vi "Z6_Beamline.ProcCases.vi"(0 "i ref in":refnum<vi>, 1 "selector":string, 2 "Data":T1, 3 "call cluster":T2={"Object"="", "Selector"="", "CallType"=enum."synchronous", "Async Object"="", "Async Selector"="", "Data Descriptor"="", "Data"=[], "Error #"=0, "Expire"=0}, 5 "error in (no error)":errorcluster) -> (14 "i ref out":refnum<vi>, 17 "answer cluster":T2={"Object"="", "Selector"="", "CallType"=enum."synchronous", "Async Object"="", "Async Selector"="", "Data Descriptor"="", "Data"=[], "Error #"=0, "Expire"=0}, 19 "error out":errorcluster)   [LabVIEW 2014, in "Z6_Beamline.lvlib"]
doc: "This method is called by a process from within the default case in the event loop. The methods of a class that are linked to events will be called from THIS method. Add your code here."
uses:
  Z6_Beamline.lvlib
  CSCore/CSSystem/CoreDefs/CoreDefs.call_type.ctl
  CSCore/BaseProcess/BaseProcess.descriptor string definition.ctl
  CSCore/CSSystem/CoreDefs/CoreDefs.rawDataType.ctl
  CSCore/CSSystem/CoreLib/CoreLib.string 2 byte array.vi
  CSCore/BaseProcess/BaseProcess.lvlib
  CSCore/CAEObj/CAEObj.lvlib
  CSCore/CSSystem/CoreLib/CoreLib.lvlib
  PH_BL-Master/PH_BL-Master.lvlib
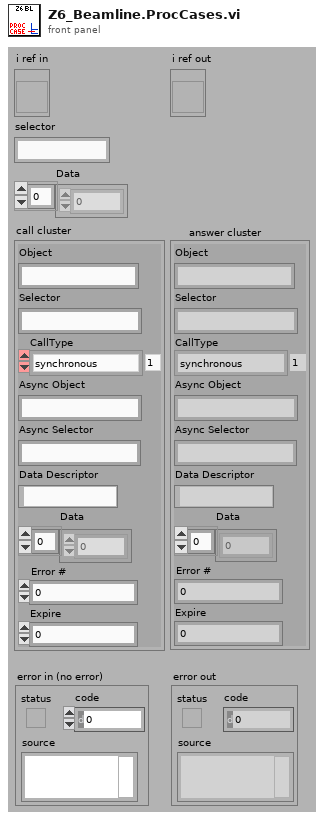
[diagram p1: front panel]
types:
  T1 = typedef "CoreDefs.rawDataType.ctl" = i8[]
  T2 = typedef "CoreDefs.call_type.ctl" = cluster{"Object":string, "Selector":string, "CallType":enum16{"simple", "synchronous", "asynchronous"}, "Async Object":string, "Async Selector":string, "Data Descriptor":T3, "Data":T1, "Error #":i32, "Expire":u32}
  T3 = typedef "BaseProcess.lvlib/BaseProcess.descriptor string definition.ctl" = string
  T4 = typedef "PH_BL-Master.lvlib/PH_BL-Master.i attribute.ctl" = cluster{"Remote controlled":bool, "Boolean Condition Service Subscriber":refnum<vi>[], "Picture Condition Service Subscriber":refnum<vi>[], "R2S":cluster{"GUI Ref":refnum<vi>, "State":bool}, "Vacua":cluster{"GUI Ref":refnum<vi>, "Limit":dbl, "Curr Value":dbl, "in range":bool}[], "O2 Inspection":cluster{"GUI Ref":refnum<vi>, "Concentration":dbl, "State":T5}[], "Boolean Status Service Subscriber":cluster{"GUI Ref":refnum<vi>, "Status":T5, "no Link?":bool, "Status Subscriber Class":T6}[], "Picture Status Service Subscriber":cluster{"GUI Ref":refnum<vi>, "Status":T5, "no Link?":bool, "Status Subscriber Class":T6}[], "6P 4Q Service Subscriber":cluster{"GUI Ref":refnum<vi>, "Selector":T7, "no Link?":bool}[], "Index of latest 6P 4Q changing Instance":i32, "Index of latest Picture Status changing Instance":i32, "Index of latest Boolean Status changing Instance":i32, "Vision ID on same Node":string, "Start Phase over?":bool, "GUI Ref Delete":refnum<vi>}
  T5 = typedef "PH_StatusHandler.lvlib/PH_StatusHandler.Status.ctl" = i16
  T6 = typedef "PH_BL-Master.lvlib/PH_BL-Master.Status Subscriber Class.ctl" = enum16{"unknown", "Switch", "BB", "6P Switch", "Switch GUI", "Switch and 6P State", "Force Sensor"}
  T7 = typedef "PH_4_Pos_Selector.lvlib/PH_4_Pos_Selector.Position Selector.ctl" = u16
  T8 = typedef "Z6_Beamline.lvlib/Z6_Beamline.i attribute.ctl" = cluster{"Subs ok GUI Refs":T9, "Refs BL Northtower":refnum<vi>[], "Refs BL Southtower":refnum<vi>[], "Refs BL 100TW COS":refnum<vi>[], "State Subsystems":cluster{"Northtower":bool, "Southtower":bool, "Frontends":bool, "100TW COS":bool}, "Z6 Beamline Status Subscriber Information":T10, "Color State PHELIX":i16}
  T9 = typedef "Z6_Beamline.lvlib/Z6_Beamline.Subsystem ok GUI Refs.ctl" = cluster{"Northtower ok":refnum<vi>, "Southtower ok":refnum<vi>, "Frontends ok":refnum<vi>, "100TW COS ok":refnum<vi>}
  T10 = typedef "Z6_Beamline.lvlib/Z6_Beamline.Status Subscriber Information.ctl" = cluster{"BL Z6 Shutter":T11, "CH 10":T11, "CH 11":T11, "ST Flip Cam":T11, "ST Flip DB":T11, "BL Z6 Dump":T11}
  T11 = typedef "PH_BL-Master.lvlib/PH_BL-Master.Status Subscriber Information.ctl" = cluster{"Index of element":i32, "Attributeset":T12}
  T12 = typedef "PH_BL-Master.lvlib/PH_BL-Master.Attribute Set.ctl" = enum16{"Boolean Status Service Subscriber", "Picture Status Service Subscriber"}
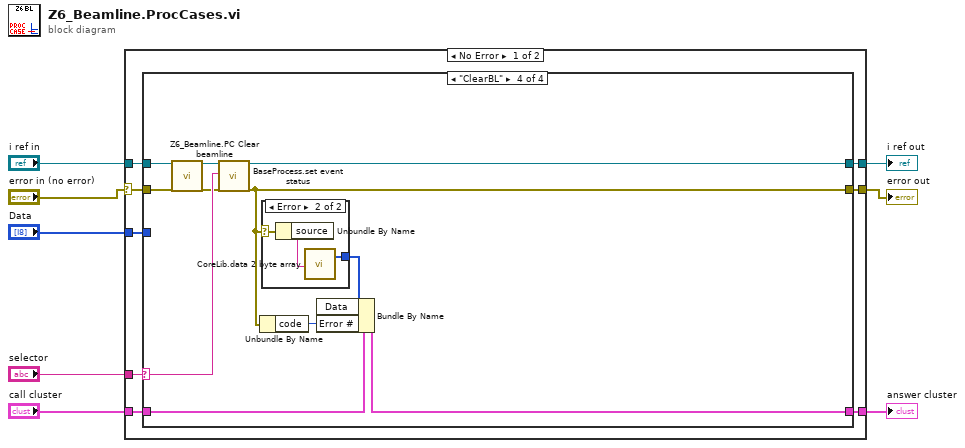
[diagram p0: block diagram]
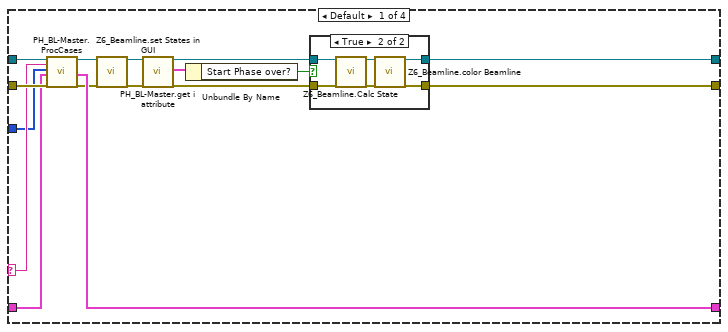
[diagram p2: hidden frame]
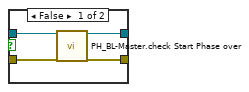
[diagram p3: hidden frame]
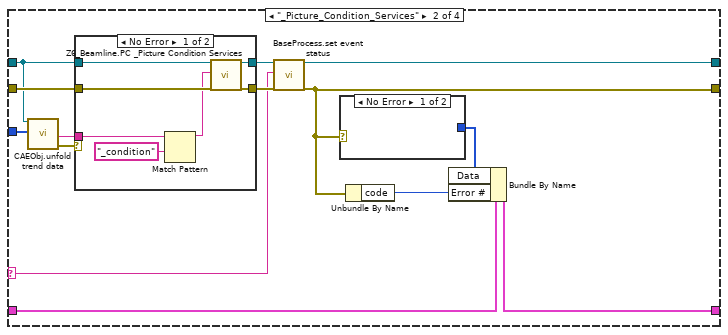
[diagram p4: hidden frame]
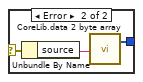
[diagram p5: hidden frame]
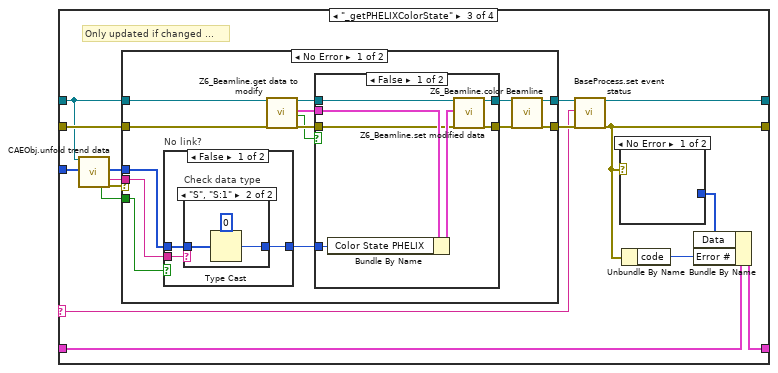
[diagram p7: hidden frame]
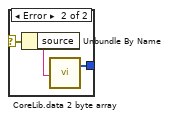
[diagram p8: hidden frame]
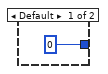
[diagram p9: hidden frame]
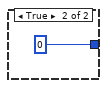
[diagram p10: hidden frame]
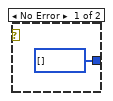
[diagram p13: hidden frame]
diagram:
  n1 = case shown="No Error" "error in (no error)" {
    selector: "error in (no error)" -> [w9 w137]
    tunnel: "selector" -> [w16 _]
    tunnel: [w15 w136] -> w7
    tunnel: "call cluster" -> [w14 w136]
    tunnel: "i ref in" -> [w13 w138]
    tunnel: [w12 w138] -> w4
    tunnel: [w11 w137] -> w3
    tunnel: "Data" -> [w10 _]
    frame No Error {
      n2 = case shown="\"ClearBL\"" w16 {
        selector: w16 -> [w29 w44 w72 w129]
        tunnel: w13 -> [w28 w53 w82 w123]
        tunnel: [w25 w47 w74 w128] -> w12
        tunnel: w14 -> [w30 w45 w71 w126]
        tunnel: [w31 w43 w70 w125] -> w15
        tunnel: w9 -> [w32 w56 w84 w124]
        tunnel: [w26 w46 w73 w127] -> w11
        tunnel: w10 -> [w27 w55 w83 _]
        frame Default {
          n3 = call "PH_BL-Master.ProcCases.vi"("i ref in"=w28, "selector"=w29, "Data"=w27, "call cluster"=w30, "error in (no error)"=w32) -> ("i ref out"=w23:refnum<vi>, "answer cluster"=w31:T2, "error out"=w24:errorcluster)  [unwired: 12 in]
          n4 = call "Z6_Beamline.set States in GUI.vi"("i ref in"=w23, "error in"=w24) -> ("i ref out"=w21:refnum<vi>, "error out"=w19:errorcluster)  [unwired: 16 in]
          n5 = call "PH_BL-Master.get i attribute.vi"("i ref in"=w21, "error in (no error)"=w19) -> ("i ref out"=w20:refnum<vi>, "i attribute"=w22:T4, "error out"=w18:errorcluster)  [unwired: 15 in]
          n6 = Unbundle By Name(w22) -> ("Start Phase over?"=w17:bool)
          n7 = case shown="True" w17 {
            tunnel: [w33 w42] -> w26
            tunnel: [w34 w41] -> w25
            tunnel: w20 -> [w35 w38]
            tunnel: w18 -> [w36 w37]
            frame False {
              n8 = call "PH_BL-Master.check Start Phase over.vi"("VI in"=w35, "error in (no error)"=w36) -> ("VI out"=w34:refnum<vi>, "error out"=w33:errorcluster)  [unwired: 16 in]
            }
            frame True {
              n9 = call "Z6_Beamline.Calc State.vi"("i ref in"=w38, "error in (no error)"=w37) -> ("i ref out"=w39:refnum<vi>, "error out"=w40:errorcluster)  [unwired: 16 in]
              n10 = call "Z6_Beamline.color Beamline.vi"("i ref in"=w39, "error in (no error)"=w40) -> ("i ref out"=w41:refnum<vi>, "error out"=w42:errorcluster)  [unwired: 16 in]
            }
          }
        }
        frame "_Picture_Condition_Services" {
          n11 = call "CAEObj.unfold trend data.vi"("i ref in"=w53, "raw trend data"=w55) -> ("serviceName"=w52:string, "error out"=w54:errorcluster)  [unwired: 9 in, 7 out]
          n12 = case shown="No Error" w54 {
            tunnel: [w63 w68] -> w49
            tunnel: w53 -> [w64 w68]
            tunnel: w56 -> [w62 w67]
            tunnel: [w61 w67] -> w48
            tunnel: w52 -> [w65 _]
            frame No Error {
              n13 = Match Pattern(string=w65, regular expression="_condition") -> (before substring=w60:string)  [unwired: 1 in, 3 out]
              n14 = call "Z6_Beamline.PC _Picture Condition Services.vi"("i ref in"=w64, "Instancename"=w60, "error IO"=w62) -> ("i ref out"=w63:refnum<vi>, "error out"=w61:errorcluster)  [unwired: 15 in]
            }
            frame Error {
            }
          }
          n15 = call "BaseProcess.set event status.vi"("i ref in"=w49, "EventStatus"=w44, "error in (no error)"=w48) -> ("i ref out"=w47:refnum<vi>, "error out"=w46:errorcluster)  [unwired: 14 in, 1 out]
          n16 = case shown="No Error" w46 {
            selector: w46 -> [_ w59]
            tunnel: [_ w57] -> w50
            frame No Error {
            }
            frame Error {
              n17 = Unbundle By Name(w59) -> ("source"=w58:string)
              n18 = call-poly "CoreLib.data 2 byte array.vi"("string"=w58) -> ("byteArray out"=w57:T1)  [unwired: 18 in]
            }
          }
          n19 = Unbundle By Name(w46) -> ("code"=w51:i32)
          n20 = Bundle By Name(cluster=w45, "Data"=w50, "Error #"=w51) -> (w43:T2)
        }
        frame "_getPHELIXColorState" {
          # "Only updated if changed ..."
          n21 = call "CAEObj.unfold trend data.vi"("i ref in"=w82, "raw trend data"=w83) -> ("no link"=w79:bool, "data"=w80:i8[], "typeDescriptor"=w69:string, "error out"=w81:errorcluster)  [unwired: 9 in, 5 out]
          n22 = case shown="No Error" w81 {
            tunnel: [w95 w120] -> w76
            tunnel: w82 -> [w101 w120]
            tunnel: w84 -> [w100 w119]
            tunnel: [w93 w119] -> w75
            tunnel: w80 -> [w90 _]
            tunnel: w79 -> [w91 _]
            tunnel: w69 -> [w89 _]
            frame No Error {
              n23 = case "No link?" shown="False" w91 {
                tunnel: [w104 i16 0] -> w88
                tunnel: w90 -> [w103 _]
                tunnel: w89 -> [w102 _]
                frame False {
                  n24 = case "Check data type" shown="\"S\", \"S:1\"" w102 {
                    tunnel: [i16 0 w106] -> w104
                    tunnel: w103 -> [_ w107]
                    frame Default {
                    }
                    frame "S", "S:1" {
                      n25 = Type Cast(type=i16 0, x=w107) -> (*(type *) &x=w106:i16)
                    }
                  }
                }
                frame True {
                }
              }
              n26 = call "Z6_Beamline.get data to modify.vi"("i ref in"=w101, "error in (no error)"=w100) -> ("i ref out"=w99:refnum<vi>, "i attribute"=w98:T8, "timed out"=w96:bool, "error out"=w97:errorcluster)  [unwired: 14 in]
              n27 = case shown="False" w96 {
                tunnel: w99 -> [w116 w118]
                tunnel: [w115 w118] -> w94
                tunnel: w98 -> [w114 _]
                tunnel: w88 -> [w112 _]
                tunnel: w97 -> [w111 w117]
                tunnel: [w110 w117] -> w92
                frame False {
                  n28 = Bundle By Name(cluster=w114, "Color State PHELIX"=w112) -> (w113:T8)
                  n29 = call "Z6_Beamline.set modified data.vi"("i ref in"=w116, "i attribute"=w113, "error in (no error)"=w111) -> ("i ref out"=w115:refnum<vi>, "error out"=w110:errorcluster)  [unwired: 15 in]
                }
                frame True {
                }
              }
              n30 = call "Z6_Beamline.color Beamline.vi"("i ref in"=w94, "error in (no error)"=w92) -> ("i ref out"=w95:refnum<vi>, "error out"=w93:errorcluster)  [unwired: 16 in]
            }
            frame Error {
            }
          }
          n31 = call "BaseProcess.set event status.vi"("i ref in"=w76, "EventStatus"=w72, "error in (no error)"=w75) -> ("i ref out"=w74:refnum<vi>, "error out"=w73:errorcluster)  [unwired: 14 in, 1 out]
          n32 = case shown="No Error" w73 {
            selector: w73 -> [_ w87]
            tunnel: [_ w85] -> w77
            frame No Error {
            }
            frame Error {
              n33 = Unbundle By Name(w87) -> ("source"=w86:string)
              n34 = call-poly "CoreLib.data 2 byte array.vi"("string"=w86) -> ("byteArray out"=w85:T1)  [unwired: 18 in]
            }
          }
          n35 = Unbundle By Name(w73) -> ("code"=w78:i32)
          n36 = Bundle By Name(cluster=w71, "Data"=w77, "Error #"=w78) -> (w70:T2)
        }
        frame "ClearBL" {
          n37 = call "Z6_Beamline.PC Clear beamline.vi"("i ref in"=w123, "error IO"=w124) -> ("i ref out"=w122:refnum<vi>, "error out"=w121:errorcluster)  [unwired: 16 in]
          n38 = call "BaseProcess.set event status.vi"("i ref in"=w122, "EventStatus"=w129, "error in (no error)"=w121) -> ("i ref out"=w128:refnum<vi>, "error out"=w127:errorcluster)  [unwired: 14 in, 1 out]
          n39 = Unbundle By Name(w127) -> ("code"=w131:i32)
          n40 = case shown="Error" w127 {
            selector: w127 -> [_ w135]
            tunnel: [T1 [] ("byteArray out") w133] -> w130
            frame No Error {
            }
            frame Error {
              n41 = Unbundle By Name(w135) -> ("source"=w134:string)
              n42 = call-poly "CoreLib.data 2 byte array.vi"("string"=w134) -> ("byteArray out"=w133:T1)  [unwired: 18 in]
            }
          }
          n43 = Bundle By Name(cluster=w126, "Data"=w130, "Error #"=w131) -> (w125:T2)
        }
      }
    }
    frame Error {
    }
  }
  "answer cluster" <- w7
  "i ref out" <- w4
  "error out" <- w3
